vi "Config Dialog.vi"(9 "Container State":T3, 10 "state in":T4={"Draw Options"={"Background Color"=16777215, "Grid Color"=13816530, "Angle Units"=enum."Radians", "Draw Solid Background"=TRUE, "Draw Grid"=TRUE, "Grid Spacing"=1.0, "AutoScale"=TRUE, "Fit to Radius"=1.0, "data row options"=[]}} caption="State", 11 "data in":T8) -> (0 "state changed?":bool, 1 "data changed?":bool, 2 "state out":T4={"Draw Options"={"Background Color"=16777215, "Grid Color"=13816530, "Angle Units"=enum."Radians", "Draw Solid Background"=TRUE, "Draw Grid"=TRUE, "Grid Spacing"=1.0, "AutoScale"=TRUE, "Fit to Radius"=1.0, "data row options"=[]}} caption="State", 3 "data out":T8)   [LabVIEW 2017, in "NI_Robotics_2D Rangefinder.xctl" / "Config Dialog.lvlib"]
uses:
  <vilib>/robotics/Controls/2D Rangefinder/_2D Rangefinder Support Files/Configuration/Config Dialog.lvlib
  <vilib>/robotics/Controls/2D Rangefinder/_2D Rangefinder Support Files/Data.ctl
  <vilib>/robotics/Controls/2D Rangefinder/_2D Rangefinder Support Files/State.ctl
  <vilib>/robotics/Controls/2D Rangefinder/2D Rangefinder Picture/Draw Options.ctl
  <vilib>/robotics/Controls/Utilities/Angle Units.ctl
  <vilib>/robotics/Controls/2D Rangefinder/2D Rangefinder Picture/Data Row Options.ctl
  <vilib>/_xctls/Container State.ctl
  <vilib>/robotics/Controls/Utilities/Color Box.ctl
  <vilib>/robotics/Controls/Utilities/Color Box_No Transparent.ctl
  <vilib>/robotics/Controls/2D Rangefinder/_2D Rangefinder Support Files/Configuration/FP Refs.ctl
  <vilib>/robotics/Controls/2D Rangefinder/2D Rangefinder Picture/NI_Robotics_2D Rangefinder Picture.lvlib
  <vilib>/robotics/Controls/2D Rangefinder/NI_Robotics_2D Rangefinder.xctl
  <vilib>/_xctls/XControlSupport.lvlib
  <vilib>/robotics/Controls/Utilities/NI_Robotics_Control Utilities.lvlib
panel:
  in  "help":bool
  in  "cancel":bool
  in  "ok":bool
  out "2D Picture":picture
  in  "line pix size":u16=5 caption="Line Width (pixels)" min=1
  in  "max line dist":dbl=inf caption="Max Line Distance" min=0.0
  in  "point pix size":u16=5 caption="Point Size (pixels)" min=1
  in  "Fit to Radius":dbl=3.0 min=0.0
  in  "autoscale":bool caption="AutoScale"
  in  "Grid Spacing":dbl=1.0 min=0.0
  in  "Angle Units":enum16{"Radians", "Degrees"}(ring)
  in  "draw lines":bool caption="Draw Lines"
  in  "lines color":T1=16711680 caption="Lines"
  in  "draw points":bool=TRUE caption="Draw Points"
  in  "points color":T1=16711680 caption="Points"
  in  "draw grid":bool=TRUE caption="Draw Grid"
  in  "grid color":T1=5865215 caption="Grid"
  in  "draw background":bool=TRUE caption="Draw Background"
  in  "bkgnd color":T2=16777226 caption="Background"
  in  "data row":i32 caption="Data Row" min=0
  in  "tab":enum32{""}(tab)
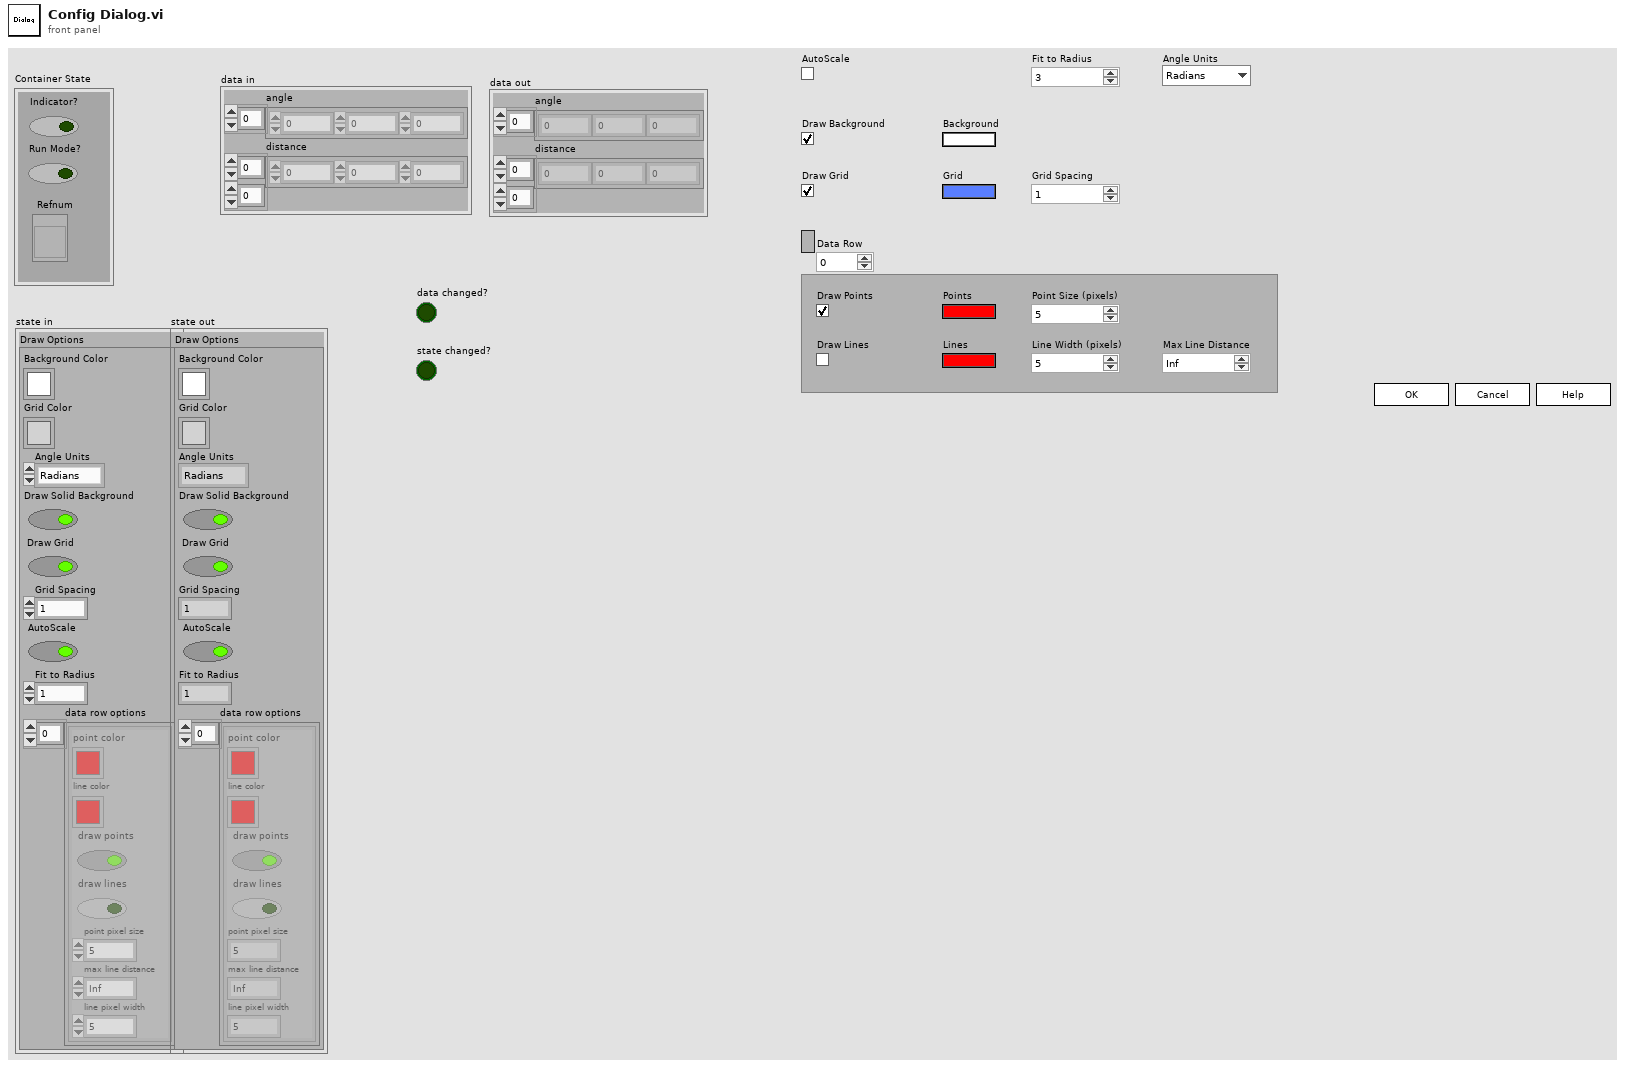
[diagram p1: front panel]
types:
  T1 = typedef "NI_Robotics_Control Utilities.lvlib/Color Box_No Transparent.ctl" = u32
  T2 = typedef "NI_Robotics_Control Utilities.lvlib/Color Box.ctl" = u32
  T3 = typedef "XControlSupport.lvlib/Container State.ctl" = cluster{"Indicator?":bool, "Run Mode?":bool, " Refnum":refnum<vi>}
  T4 = typedef "NI_Robotics_2D Rangefinder.xctl/State.ctl" = cluster{"Draw Options":T5}
  T5 = typedef "NI_Robotics_2D Rangefinder Picture.lvlib/Draw Options.ctl" = cluster{"Background Color":u32, "Grid Color":u32, "Angle Units":T6, "Draw Solid Background":bool, "Draw Grid":bool, "Grid Spacing":dbl, "AutoScale":bool, "Fit to Radius":dbl, "data row options":T7[]}
  T6 = typedef "NI_Robotics_Control Utilities.lvlib/Angle Units.ctl" = enum16{"Radians", "Degrees"}
  T7 = typedef "NI_Robotics_2D Rangefinder Picture.lvlib/Data Row Options.ctl" = cluster{"point color":u32, "line color":u32, "draw points":bool, "draw lines":bool, "point pixel size":u16, "max line distance":dbl, "line pixel width":u16}
  T8 = typedef "NI_Robotics_2D Rangefinder.xctl/Data.ctl" = cluster{"angle":dbl[], "distance":dbl[][]}
  T9 = typedef "NI_Robotics_2D Rangefinder.xctl/Config Dialog.lvlib/FP Refs.ctl" = cluster{"dialog VI":refnum<vi>, "picture":refnum<vi>, "bkgnd color":refnum<vi>, "grid color":refnum<vi>, "Angle Units":refnum<vi>, "draw background":refnum<vi>, "draw grid":refnum<vi>, "Grid Spacing":refnum<vi>, "autoscale":refnum<vi>, "Fit to Radius":refnum<vi>, "data row":refnum<vi>, "points color":refnum<vi>, "lines color":refnum<vi>, "draw points":refnum<vi>, "draw lines":refnum<vi>, "point pix size":refnum<vi>, "max line dist":refnum<vi>, "line pix size":refnum<vi>}
  T10 = typedef "NI_Robotics_2D Rangefinder Picture.lvlib/Rangefinder Data.ctl" = cluster{"Angle":dbl[], "Distance":dbl[][]}
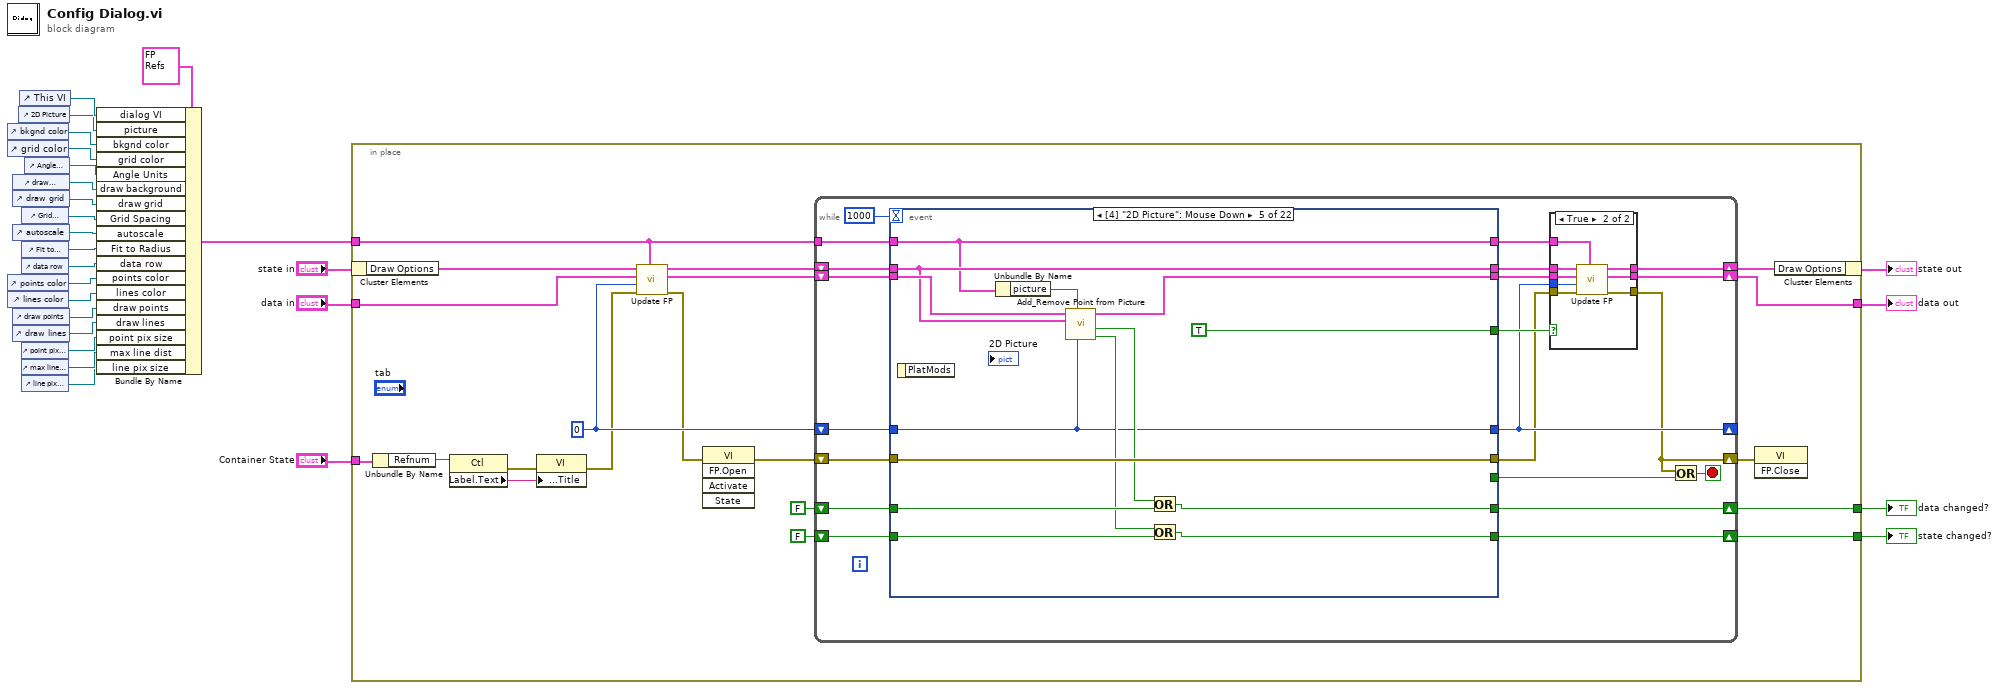
[diagram p0: block diagram]
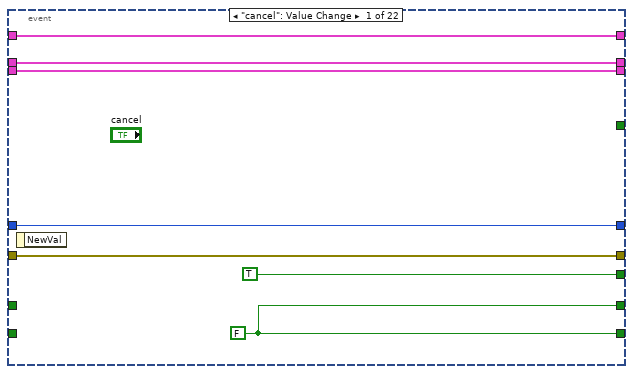
[diagram p3: hidden frame]
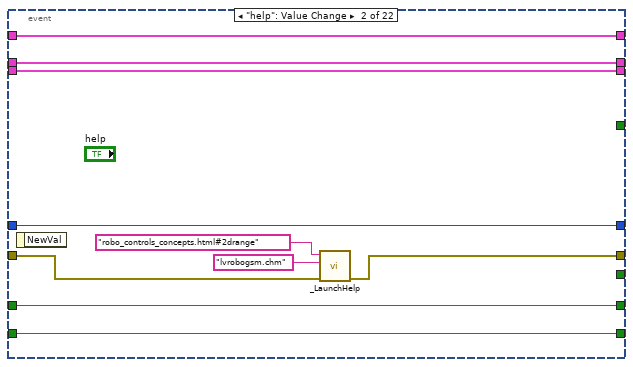
[diagram p4: hidden frame]
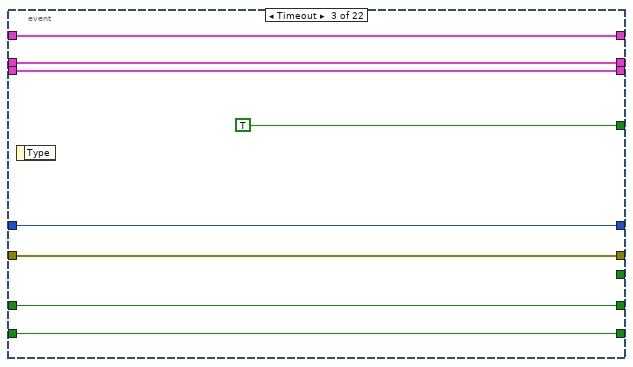
[diagram p5: hidden frame]
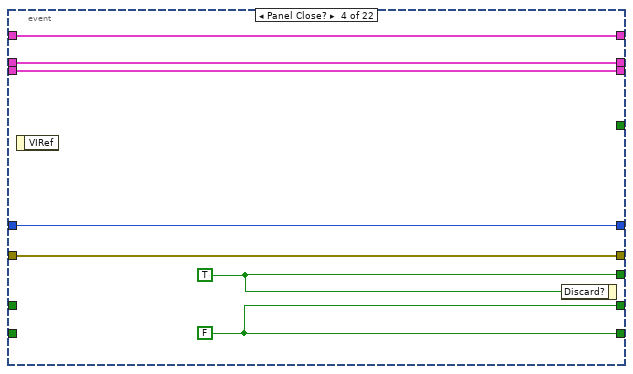
[diagram p6: hidden frame]
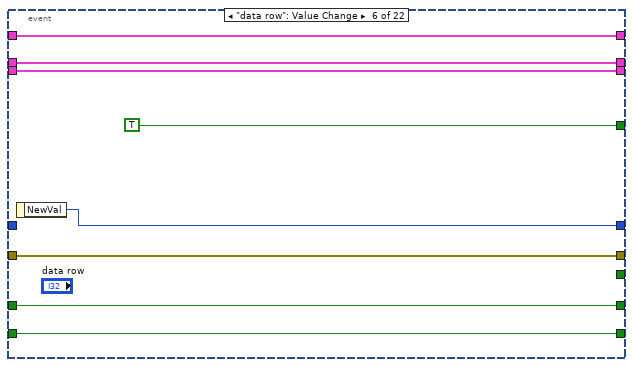
[diagram p7: hidden frame]
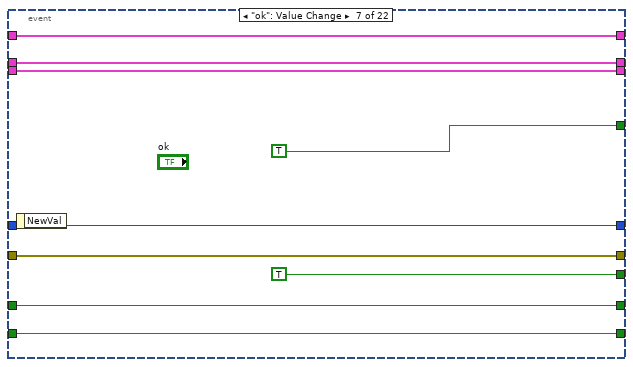
[diagram p8: hidden frame]
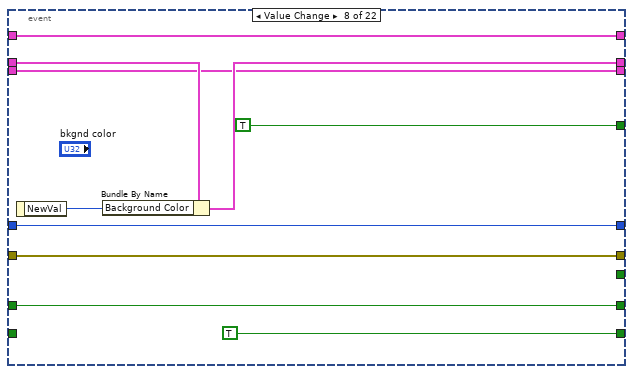
[diagram p9: hidden frame]
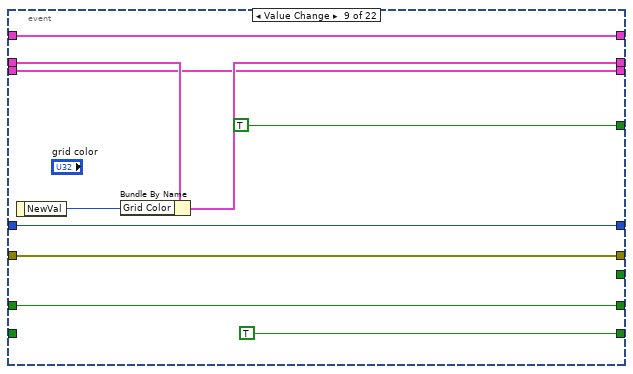
[diagram p10: hidden frame]
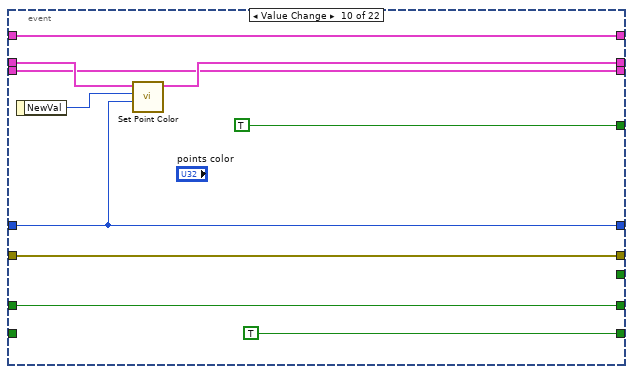
[diagram p11: hidden frame]
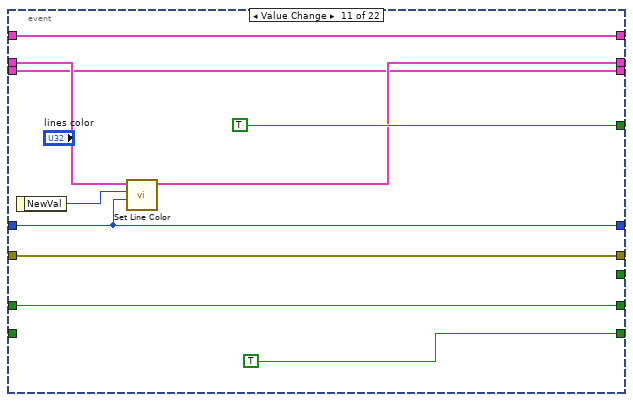
[diagram p12: hidden frame]
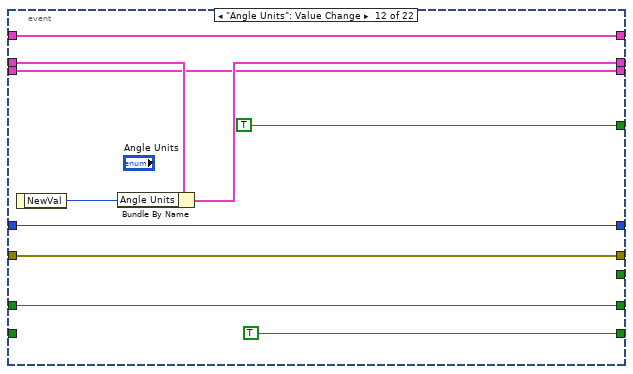
[diagram p13: hidden frame]
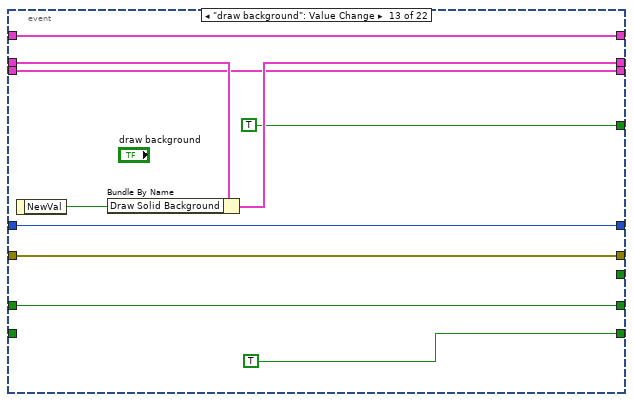
[diagram p14: hidden frame]
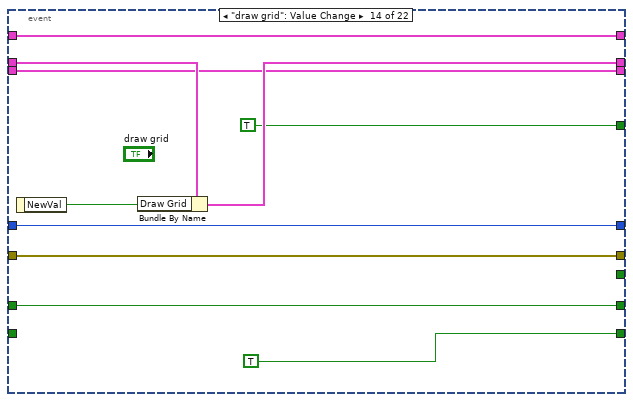
[diagram p15: hidden frame]
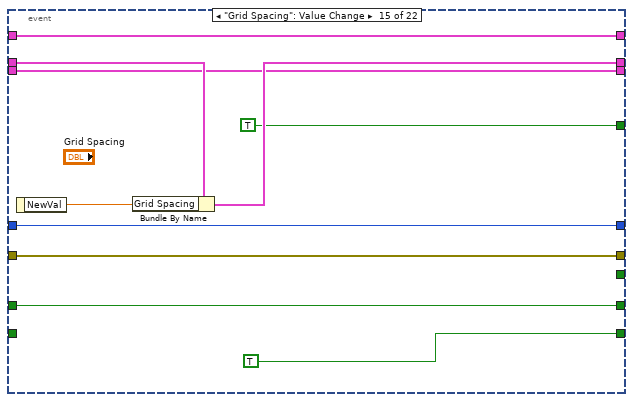
[diagram p16: hidden frame]
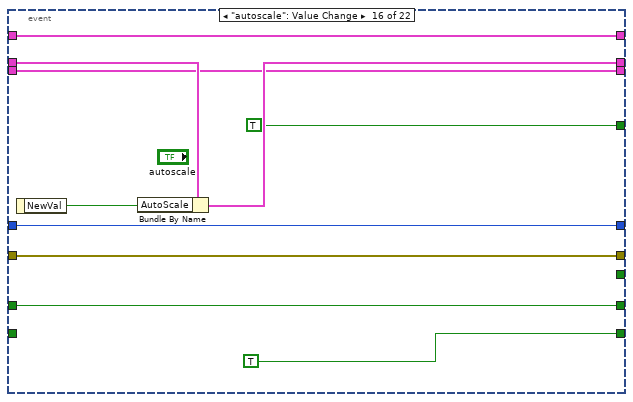
[diagram p17: hidden frame]
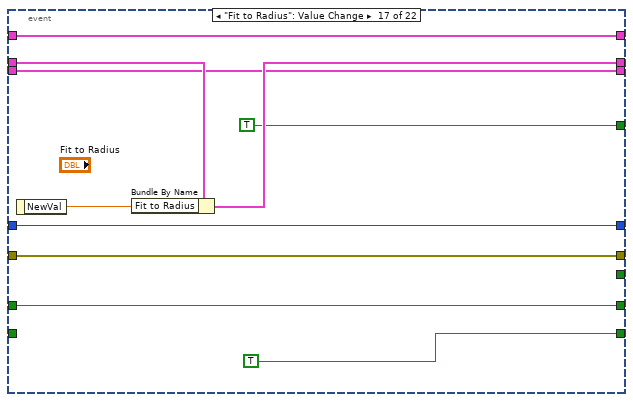
[diagram p18: hidden frame]
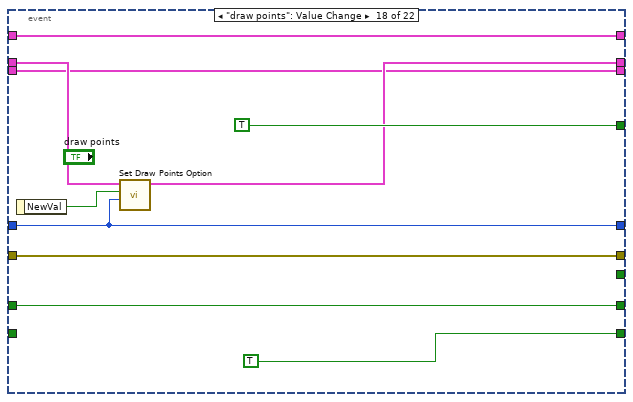
[diagram p19: hidden frame]
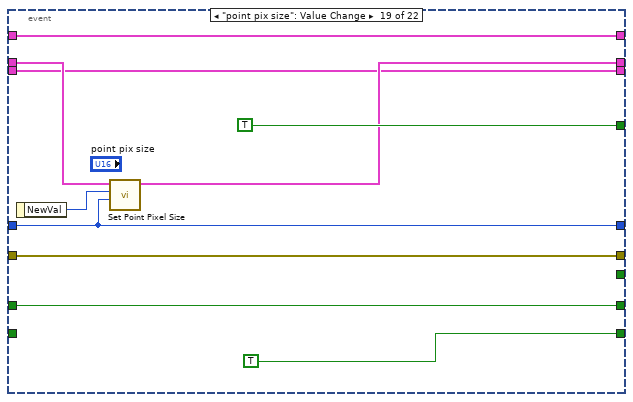
[diagram p20: hidden frame]
diagram:
  n1 = control-ref of="bkgnd color"() -> (w20:refnum<vi>)
  n2 = control-ref of="grid color"() -> (w3:refnum<vi>)
  n3 = control-ref of="points color"() -> (w2:refnum<vi>)
  n4 = control-ref of="lines color"() -> (w1:refnum<vi>)
  n5 = control-ref of="draw background"() -> (w18:refnum<vi>)
  n6 = control-ref of="draw grid"() -> (w17:refnum<vi>)
  n7 = control-ref of="autoscale"() -> (w15:refnum<vi>)
  n8 = control-ref of="draw points"() -> (w13:refnum<vi>)
  n9 = control-ref of="draw lines"() -> (w12:refnum<vi>)
  n10 = control-ref of="2D Picture"() -> (w6:refnum<vi>)
  n11 = control-ref of="This VI"() -> (w7:refnum<vi>)
  n12 = control-ref of="Grid Spacing"() -> (w16:refnum<vi>)
  n13 = control-ref of="Fit to Radius"() -> (w14:refnum<vi>)
  n14 = control-ref of="data row"() -> (w4:refnum<vi>)
  n15 = control-ref of="point pix size"() -> (w11:refnum<vi>)
  n16 = control-ref of="max line dist"() -> (w10:refnum<vi>)
  n17 = control-ref of="line pix size"() -> (w9:refnum<vi>)
  n18 = control-ref of="Angle Units"() -> (w19:refnum<vi>)
  n19 = Bundle By Name(cluster=T9 {"dialog VI"=refnum, "picture"=refnum, "bkgnd color"=refnum, "grid color"=refnum, "Angle Units"=refnum, "draw background"=refnum, "draw grid"=refnum, "Grid Spacing"=refnum, "autoscale"=refnum, "Fit to Radius"=refnum, "data row"=refnum, "points color"=refnum, "lines color"=refnum, "draw points"=refnum, "draw lines"=refnum, "point pix size"=refnum, "max line dist"=refnum, "line pix size"=refnum} ("FP refs"), "dialog VI"=w7, "picture"=w6, "bkgnd color"=w20, "grid color"=w3, "Angle Units"=w19, "draw background"=w18, "draw grid"=w17, "Grid Spacing"=w16, "autoscale"=w15, "Fit to Radius"=w14, "data row"=w4, "points color"=w2, "lines color"=w1, "draw points"=w13, "draw lines"=w12, "point pix size"=w11, "max line dist"=w10, "line pix size"=w9) -> (w8:T9)
  n20 = in-place {
    in-place-border: "Container State" -> [w45]
    in-place-border: "data in" -> [w44]
    in-place-border: [w41] -> w23
    in-place-border: [w40] -> w22
    in-place-border: w8 -> [w28]
    in-place-border: [w38] -> w5
    w39 = 0 ("data row index")
    n21 = in-place-cluster #1("state in") -> ("Draw Options"=w47:T5)
    n22 = Unbundle By Name(w45) -> ("Refnum"=w35:refnum<vi>)
    n23 = property class="Ctl"(reference=w35) -> (error out=w34:errorcluster, "Label.Text"=w36:string)  [unwired: 1 in, 1 out]
    n24 = property class="VI"(error in=w34, "Front Panel.Title"=w36) -> (error out=w33:errorcluster)  [unwired: 1 in, 1 out]
    n25 = call <vilib>:"Update FP.vi"("FP refs"=w28, "error in (no error)"=w33, "data row index"=w39, "rangefinder data in"=w44, "draw options in"=w47) -> ("error out"=w37:errorcluster, "rangefinder data out"=w43:T10, "draw options out"=w46:T5)  [unwired: 4 in]
    n26 = invoke class="VI" method="FP.Open"(error in=w37) -> (error out=w32:errorcluster)  [unwired: 4 in, 4 out]
    n27 = while {
      shift-right: [w54] -> w42
      shift-left: w46 -> [w67]
      shift-right: [w52] -> w29
      shift-left: w32 -> [w62]
      shift-right: [w64] -> w41
      shift-left: FALSE -> [w66]
      shift-right: [w63] -> w40
      shift-left: FALSE -> [w65]
      shift-right: [w56] -> _
      shift-left: w39 -> [w58]
      shift-right: [w57] -> w38
      shift-left: w43 -> [w51]
      tunnel: w28 -> [w49]
      stop <- w61 stop-if-true
      n28 = event shown="[4] \"2D Picture\": Mouse Down" {
        selector: _ -> [_ _ _ _ _ _ _ _ _ _ _ _ _ _ _ _ _ _ _ _ _ _]
        dyn-events: _ -> [_ _ _ _ _ _ _ _ _ _ _ _ _ _ _ _ _ _ _ _ _ _]
        timeout: 1000 -> [_ _ _ _ _ _ _ _ _ _ _ _ _ _ _ _ _ _ _ _ _ _]
        tunnel: w67 -> [w86 w94 w102 w111 w122 w128 w140 w149 w159 w168 w178 w189 w199 w209 w219 w229 w239 w248 w258 w268 w278 w288]
        tunnel: w66 -> [_ w96 w104 _ w120 w133 w142 w152 w162 w172 w182 w192 w202 w212 w222 w232 w242 w252 w262 w272 w282 w292]
        tunnel: w65 -> [_ w95 w103 _ w117 w132 w141 _ _ _ _ _ _ _ _ _ _ _ _ _ _ _]
        tunnel: [w83 w96 w104 w108 w119 w133 w142 w152 w162 w172 w182 w192 w202 w212 w222 w232 w242 w252 w262 w272 w282 w292] -> w64
        tunnel: [w83 w95 w103 w108 w116 w132 w141 TRUE TRUE TRUE TRUE TRUE TRUE TRUE TRUE TRUE TRUE TRUE TRUE TRUE TRUE TRUE] -> w63
        tunnel: [w86 w94 w102 w111 w122 w128 w140 w148 w158 w167 w177 w188 w198 w208 w218 w228 w238 w247 w257 w265 w277 w287] -> w55
        tunnel: w62 -> [w85 w90 w101 w110 w125 w131 w139 w151 w161 w171 w181 w191 w201 w211 w221 w231 w241 w251 w261 w271 w281 w291]
        tunnel: [w85 w89 w101 w110 w125 w131 w139 w151 w161 w171 w181 w191 w201 w211 w221 w231 w241 w251 w261 w271 w281 w291] -> w53
        tunnel: [_ _ TRUE _ TRUE ("update picture (F)") TRUE ("update picture (F)") TRUE TRUE TRUE TRUE TRUE TRUE TRUE TRUE TRUE TRUE TRUE TRUE TRUE TRUE TRUE TRUE] -> w60
        tunnel: [TRUE _ _ w109 _ _ TRUE _ _ _ _ _ _ _ _ _ _ _ _ _ _ _] -> w59
        tunnel: [w82 w93 w99 w107 w113 w130 w136 w145 w155 w165 w175 w185 w195 w205 w215 w225 w235 w245 w255 w266 w275 w285] -> w56
        tunnel: w58 -> [w82 w93 w99 w107 w113 _ w136 w145 w155 w165 w175 w185 w195 w205 w215 w225 w235 w245 w255 w266 w275 w285]
        tunnel: w51 -> [w81 w88 w98 w106 w124 w127 w135 w144 w154 w164 w174 w184 w194 w204 w214 w224 w234 w244 w254 w264 w274 w284]
        tunnel: [w81 w88 w98 w106 w123 w127 w135 w144 w154 w164 w174 w184 w194 w204 w214 w224 w234 w244 w254 w264 w274 w284] -> w50
        tunnel: w49 -> [w80 w87 w97 w105 w115 w126 w134 w143 w153 w163 w173 w183 w193 w203 w213 w223 w233 w243 w253 w263 w273 w283]
        tunnel: [w80 w87 w97 w105 w115 w126 w134 w143 w153 w163 w173 w183 w193 w203 w213 w223 w233 w243 w253 w263 w273 w283] -> w48
        event "cancel": Value Change {
          w83 = FALSE
          n29 = event-data() -> ()  [unwired: 1 in, 1 out]
        }
        event "help": Value Change {
          n30 = event-data() -> ()  [unwired: 1 in, 1 out]
          n31 = call <helpdir>:"_LaunchHelp.vi"("error in (no error)"=w90, "CHM or HLP filename (lvdialog.chm)"="lvrobogsm.chm", "HTML filename"="robo_controls_concepts.html#2drange") -> ("error out"=w89:errorcluster)  [unwired: 4 out]
        }
        event Timeout {
          n32 = event-data() -> ()  [unwired: 1 in, 1 out]
        }
        event Panel Close? {
          w108 = FALSE
          w109 = TRUE
          n33 = event-data() -> ()  [unwired: 1 in, 1 out]
          n34 = event-data("Discard?"=w109) -> ()  [unwired: 1 in, 1 out]
        }
        event "2D Picture": Mouse Down {
          n35 = event-data() -> ()  [unwired: 1 in, 1 out]
          n36 = Unbundle By Name(w115) -> ("picture"=w114:refnum<vi>)
          n37 = call <vilib>:"Add_Remove Point from Picture.vi"("row index (0)"=w113, "2D Picture"=w114, "draw options"=w122, "data in"=w124) -> ("state changed?"=w118:bool, "data changed?"=w121:bool, "data out"=w123:T10)  [unwired: 5 in]
          n38 = Or(x=w121, y=w120) -> (x .or. y?=w119:bool)
          n39 = Or(x=w118, y=w117) -> (x .or. y?=w116:bool)
        }
        event "data row": Value Change {
          n40 = event-data() -> ("NewVal"=w130:i32)  [unwired: 1 in]
        }
        event "ok": Value Change {
          n41 = event-data() -> ()  [unwired: 1 in, 1 out]
        }
        event Value Change {
          n42 = event-data() -> ("NewVal"=w150:T2)  [unwired: 1 in]
          n43 = Bundle By Name(cluster=w149, "Background Color"=w150) -> (w148:T5)
        }
        event Value Change {
          n44 = event-data() -> ("NewVal"=w160:T1)  [unwired: 1 in]
          n45 = Bundle By Name(cluster=w159, "Grid Color"=w160) -> (w158:T5)
        }
        event Value Change {
          n46 = event-data() -> ("NewVal"=w166:T1)  [unwired: 1 in]
          n47 = call <vilib>:"Set Point Color.vi"("data row index"=w165, "point color"=w166, "draw options in"=w168) -> ("draw options out"=w167:T5)  [unwired: 8 in]
        }
        event Value Change {
          n48 = event-data() -> ("NewVal"=w176:T1)  [unwired: 1 in]
          n49 = call <vilib>:"Set Line Color.vi"("data row index"=w175, "line color"=w176, "draw options in"=w178) -> ("draw options out"=w177:T5)  [unwired: 8 in]
        }
        event "Angle Units": Value Change {
          n50 = event-data() -> ("NewVal"=w190:enum16{"Radians", "Degrees"})  [unwired: 1 in]
          n51 = Bundle By Name(cluster=w189, "Angle Units"=w190) -> (w188:T5)
        }
        event "draw background": Value Change {
          n52 = event-data() -> ("NewVal"=w200:bool)  [unwired: 1 in]
          n53 = Bundle By Name(cluster=w199, "Draw Solid Background"=w200) -> (w198:T5)
        }
        event "draw grid": Value Change {
          n54 = event-data() -> ("NewVal"=w210:bool)  [unwired: 1 in]
          n55 = Bundle By Name(cluster=w209, "Draw Grid"=w210) -> (w208:T5)
        }
        event "Grid Spacing": Value Change {
          n56 = event-data() -> ("NewVal"=w220:dbl)  [unwired: 1 in]
          n57 = Bundle By Name(cluster=w219, "Grid Spacing"=w220) -> (w218:T5)
        }
        event "autoscale": Value Change {
          n58 = event-data() -> ("NewVal"=w230:bool)  [unwired: 1 in]
          n59 = Bundle By Name(cluster=w229, "AutoScale"=w230) -> (w228:T5)
        }
        event "Fit to Radius": Value Change {
          n60 = event-data() -> ("NewVal"=w240:dbl)  [unwired: 1 in]
          n61 = Bundle By Name(cluster=w239, "Fit to Radius"=w240) -> (w238:T5)
        }
        event "draw points": Value Change {
          n62 = event-data() -> ("NewVal"=w246:bool)  [unwired: 1 in]
          n63 = call <vilib>:"Set Draw Points Option.vi"("data row index"=w245, "draw points"=w246, "draw options in"=w248) -> ("draw options out"=w247:T5)  [unwired: 8 in]
        }
        event "point pix size": Value Change {
          n64 = event-data() -> ("NewVal"=w256:u16)  [unwired: 1 in]
          n65 = call <vilib>:"Set Point Pixel Size.vi"("data row index"=w255, "point pixel size"=w256, "draw options in"=w258) -> ("draw options out"=w257:T5)  [unwired: 8 in]
        }
        event "draw lines": Value Change {
          n66 = event-data() -> ("NewVal"=w267:bool)  [unwired: 1 in]
          n67 = call <vilib>:"Set Draw Lines Option.vi"("data row index"=w266, "draw lines"=w267, "draw options in"=w268) -> ("draw options out"=w265:T5)  [unwired: 8 in]
        }
        event "max line dist": Value Change {
          n68 = event-data() -> ("NewVal"=w276:dbl)  [unwired: 1 in]
          n69 = call <vilib>:"Set Max Line Distance.vi"("data row index"=w275, "max line distance"=w276, "draw options in"=w278) -> ("draw options out"=w277:T5)  [unwired: 8 in]
        }
        event "line pix size": Value Change {
          n70 = event-data() -> ("NewVal"=w286:u16)  [unwired: 1 in]
          n71 = call <vilib>:"Set Line Pixel Width.vi"("data row index"=w285, "line pixel width"=w286, "draw options in"=w288) -> ("draw options out"=w287:T5)  [unwired: 8 in]
        }
      }
      n72 = case shown="True" w60 {
        tunnel: w55 -> [w70 w79]
        tunnel: w50 -> [w71 w78]
        tunnel: [w71 w77] -> w57
        tunnel: w56 -> [_ w76]
        tunnel: [w70 w73] -> w54
        tunnel: w53 -> [w69 w75]
        tunnel: [w69 w74] -> w52
        tunnel: w48 -> [_ w72]
        frame False {
        }
        frame True {
          n73 = call <vilib>:"Update FP.vi"("FP refs"=w72, "error in (no error)"=w75, "data row index"=w76, "rangefinder data in"=w78, "draw options in"=w79) -> ("error out"=w74:errorcluster, "rangefinder data out"=w77:T10, "draw options out"=w73:T5)  [unwired: 4 in]
        }
      }
      n74 = Or(x=w52, y=w59) -> (x .or. y?=w61:bool)
    }
    n75 = invoke class="VI" method="FP.Close"(error in=w29) -> ()  [unwired: 2 in, 3 out]
    n76 = in-place-cluster #1("Draw Options"=w42) -> (→"state out":T4)
  }
  "data out" <- w5
  "data changed?" <- w23
  "state changed?" <- w22
